vi "Set RT System Clock by NTP Server.vi"(2 "error in (no error)":errorcluster, 3 "Time Server IP":string="132.163.4.102") -> (0 "error out":errorcluster, 1 "Time Set":timestamp)   [LabVIEW 2013]
uses:
  <vilib>/Utility/miscctls.llb/LVDateTimeRec.ctl
  <vilib>/nisyscfg/nisyscfg.lvlib
panel:
  out "Time Set?":bool
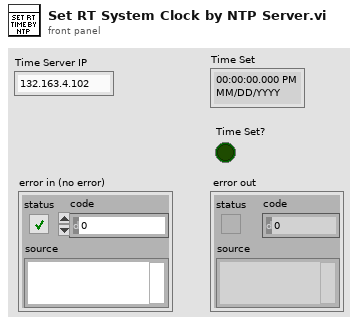
[diagram p1: front panel]
types:
  T1 = typedef "LVDateTimeRec.ctl" = cluster{"fractional second":dbl, "second":i32, "minute":i32, "hour":i32, "day of month":i32, "month":i32, "year":i32, "day of week":i32, "day of year":i32, "DST":i32}
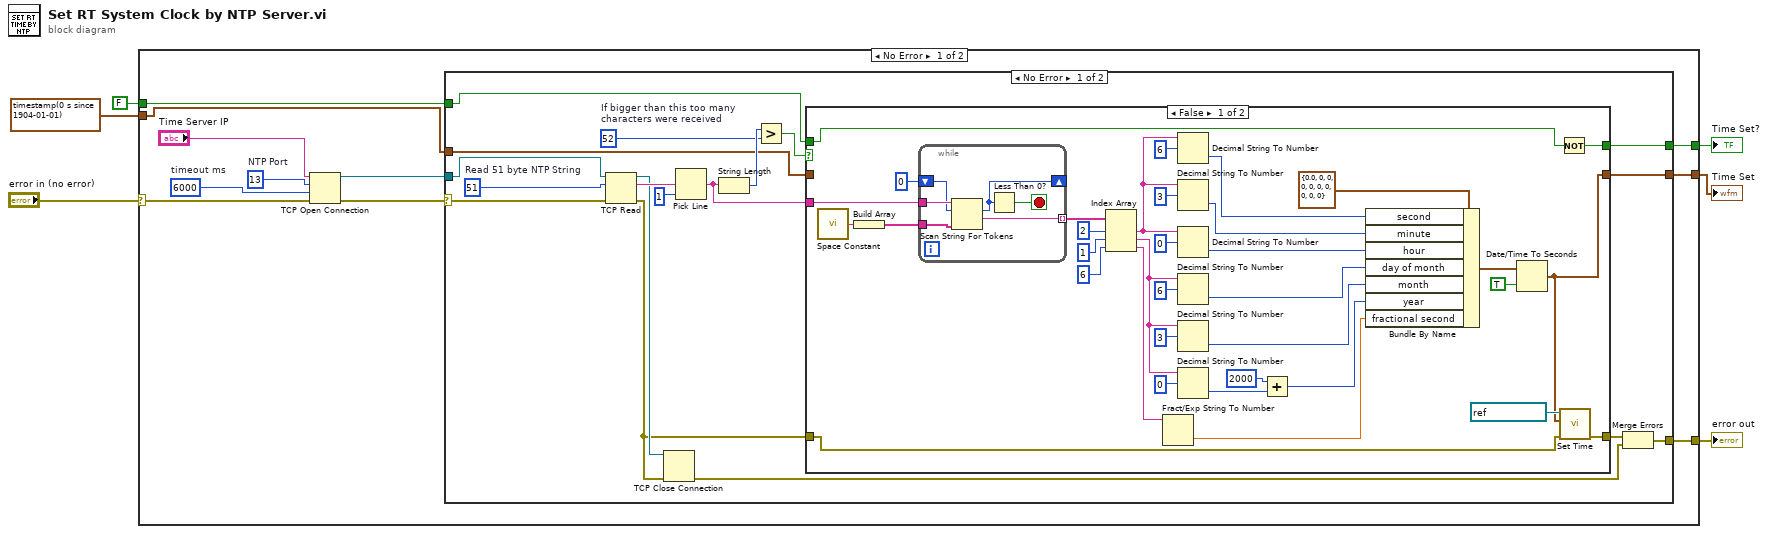
[diagram p0: block diagram]
diagram:
  n1 = case shown="No Error" "error in (no error)" {
    selector: "error in (no error)" -> [w10 w85]
    tunnel: [w12 w85] -> w6
    tunnel: [w11 w84] -> w3
    tunnel: timestamp(0 s since 1904-01-01) ("Time Set") -> [w9 w84]
    tunnel: [w8 w83] -> w2
    tunnel: FALSE -> [w7 w83]
    frame No Error {
      w15 = 6000  # timeout ms
      w16 = u16 13  # NTP Port
      n2 = TCP Open Connection(address="Time Server IP", remote port or service name=w16, timeout ms (60000)=w15, error in (no error)=w10) -> (connection ID=w17:refnum<k5>, error out=w14:errorcluster)  [unwired: 1 in]
      n3 = case shown="No Error" w14 {
        selector: w14 -> [w27 w82]
        tunnel: w17 -> [w34 _]
        tunnel: [w22 w82] -> w12
        tunnel: [w24 w81] -> w11
        tunnel: w9 -> [w20 w81]
        tunnel: [w19 w80] -> w8
        tunnel: w7 -> [w18 w80]
        frame No Error {
          w28 = 52  # If bigger than this too many characters were received
          w35 = 51  # Read 51 byte NTP String
          n4 = TCP Read(connection ID=w34, bytes to read=w35, error in (no error)=w27) -> (connection ID out=w26:refnum<k5>, data out=w32:string, error out=w23:errorcluster)  [unwired: 2 in]
          n5 = TCP Close Connection(connection ID=w26, error in (no error)=w23) -> (error out=w21:errorcluster)  [unwired: 1 in, 1 out]
          n6 = Pick Line(multi-line string=w32, line index=1) -> (output string=w31:string)  [unwired: 1 in]
          n7 = String Length(string=w31) -> (length=w30:i32)
          n8 = Greater?(x=w30, y=w28) -> (0:w29:bool)
          n9 = case shown="False" w29 {
            tunnel: w31 -> [w41 _]
            tunnel: w23 -> [w52 w79]
            tunnel: [w51 w79] -> w25
            tunnel: [w43 w78] -> w24
            tunnel: w20 -> [_ w78]
            tunnel: [w37 w77] -> w19
            tunnel: w18 -> [w36 w77]
            frame False {
              n10 = call <vilib>:"Space Constant.vi"() -> ("String"=w40:string)
              n11 = Build Array(w40) -> (w39:string[])
              n12 = while {
                tunnel: w41 -> [w76]
                shift-right: [w71] -> _
                shift-left: 0 ("offset past token") -> [w75]
                tunnel: [w74] -> w42 mode=indexing
                tunnel: w39 -> [w73]
                stop <- w72 stop-if-true
                n13 = Scan String For Tokens(6:w73, 8:w75, 9:w76) -> (1:w74:string, 2:w71:i32)  [unwired: 3 in, 2 out]
                n14 = Less Than 0?(x=w71) -> (x < 0?=w72:bool)
              }
              n15 = Index Array(array=w42, index #1=2 ("index"), index #2=1 ("index"), index #3=6 ("index")) -> (element #1=w47:string, element #2=w46:string, element #3=w45:string)
              n16 = Fract/Exp String To Number(string=w45) -> (number=w68:dbl)  [unwired: 3 in, 1 out]
              n17 = Decimal String To Number(string=w47, offset=6) -> (number=w57:i32)  [unwired: 1 in, 1 out]
              n18 = Decimal String To Number(string=w47, offset=3) -> (number=w61:i32)  [unwired: 1 in, 1 out]
              n19 = Decimal String To Number(string=w47, offset=0) -> (number=w59:i32)  [unwired: 1 in, 1 out]
              n20 = Decimal String To Number(string=w46, offset=6) -> (number=w63:i32)  [unwired: 1 in, 1 out]
              n21 = Decimal String To Number(string=w46, offset=3) -> (number=w65:i32)  [unwired: 1 in, 1 out]
              n22 = Decimal String To Number(string=w46, offset=0) -> (number=w67:i32)  [unwired: 1 in, 1 out]
              n23 = Add(x=2000, y=w67) -> (x+y=w69:i32)
              n24 = Bundle By Name(cluster=T1 {"fractional second"=0.0, "second"=0, "minute"=0, "hour"=0, "day of month"=0, "month"=0, "year"=0, "day of week"=0, "day of year"=0, "DST"=0} ("date time rec"), "second"=w57, "minute"=w61, "hour"=w59, "day of month"=w63, "month"=w65, "year"=w69, "fractional second"=w68) -> (w54:T1)
              n25 = Date/Time To Seconds(1:TRUE ("is UTC (F)"), 2:w54) -> (0:w43:timestamp)
              n26 = Not(x=w36) -> (.not. x?=w37:bool)
              n27 = call <vilib>:"Set Time.vi"("error in (no error)"=w52, "time"=w43, "session in (localhost)"=refnum<k21> "localhost") -> ("error out"=w51:errorcluster)  [unwired: 5 in, 3 out]
            }
            frame True {
            }
          }
          n28 = Merge Errors(w25, w21) -> (w22:errorcluster)
        }
        frame Error {
          # "Network Error Do Nothing"
        }
      }
    }
    frame Error {
    }
  }
  "error out" <- w6
  "Time Set" <- w3
  "Time Set?" <- w2
